vi "Exercise 4-1.vi"(0 "Current Temp":dbl, 1 "Max Temp":dbl, 2 "Min Temp 2":dbl, 3 "error in (no error)":errorcluster) -> (8 "Warning Text":string, 9 "Warning?":bool, 10 "error out":errorcluster)   [LabVIEW 2014]
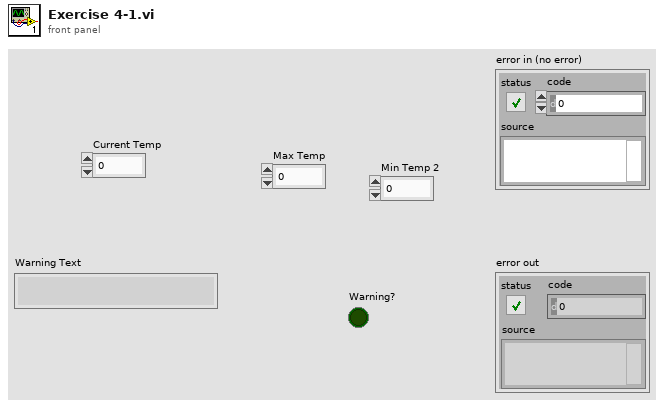
[diagram p1: front panel]
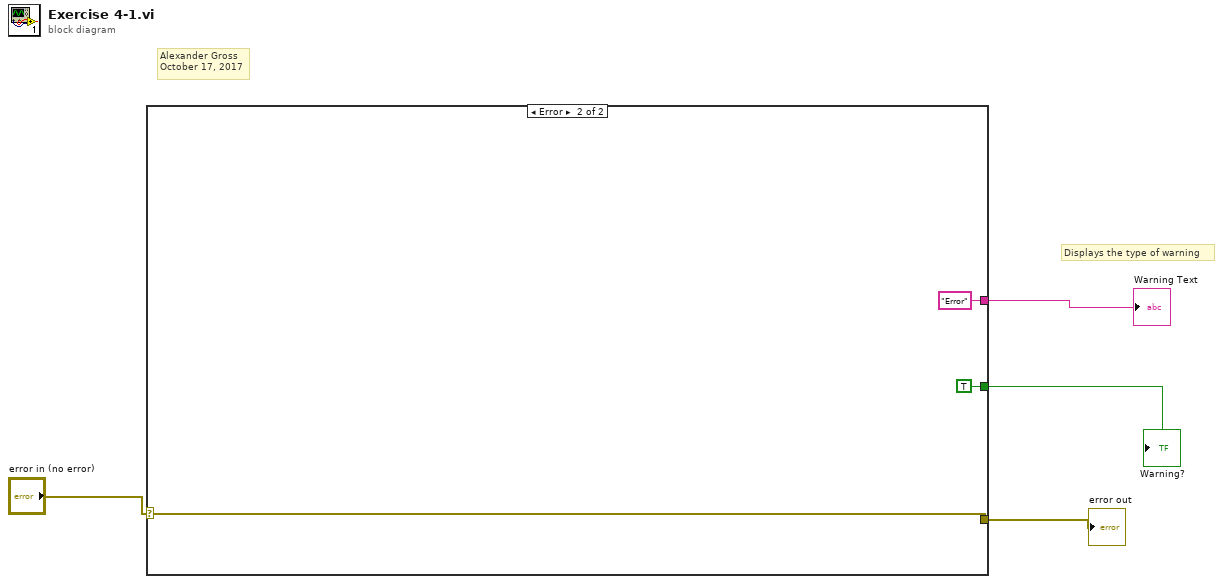
[diagram p0: block diagram]
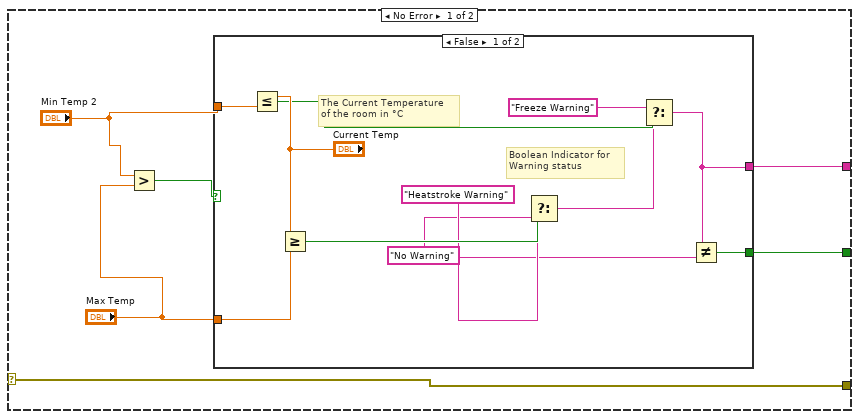
[diagram p2: hidden frame]
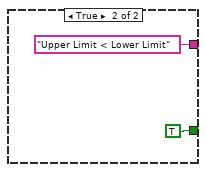
[diagram p3: hidden frame]
diagram:
  # "Alexander Gross\nOctober 17, 2017"
  # "Displays the type of warning"
  n1 = case shown="Error" "error in (no error)" {
    selector: "error in (no error)" -> [w5 w26]
    tunnel: [w10 "Error"] -> w4
    tunnel: [w9 TRUE] -> w3
    tunnel: [w5 w26] -> w1
    frame No Error {
      n2 = Greater?(x="Min Temp 2", y="Max Temp") -> (0:w6:bool)
      n3 = case shown="False" w6 {
        tunnel: [w14 "Upper Limit < Lower Limit"] -> w10
        tunnel: [w13 TRUE] -> w9
        tunnel: "Min Temp 2" -> [w12 _]
        tunnel: "Max Temp" -> [w11 _]
        frame False {
          w15 = "No Warning"
          # "Boolean Indicator for \nWarning status"
          # "The Current Temperature \nof the room in °C"
          n4 = Less Or Equal?(x="Current Temp", y=w12) -> (x <= y?=w18:bool)
          n5 = Greater Or Equal?(x="Current Temp", y=w11) -> (x >= y?=w20:bool)
          n6 = Select(t="Heatstroke Warning", s=w20, f=w15) -> (s? t:f=w16:string)
          n7 = Select(t="Freeze Warning", s=w18, f=w16) -> (s? t:f=w14:string)
          n8 = Not Equal?(x=w14, y=w15) -> (x != y?=w13:bool)
        }
        frame True {
        }
      }
    }
    frame Error {
    }
  }
  "Warning Text" <- w4
  "Warning?" <- w3
  "error out" <- w1
